vi "Program Single.vi"(8 "error in (no error)":errorcluster, 9 "Micro":string, 10 "Positions":u32, 11 "Program Driver in":refnum<class "Program Driver.lvclass">) -> (0 "error out":errorcluster, 1 "Fail Codes":string, 2 "Tests Passed":bool, 3 "Program Driver out":refnum<class "Program Driver.lvclass">)   [LabVIEW 2015, in "Program Driver.lvclass"]
uses:
  Program Driver.lvclass
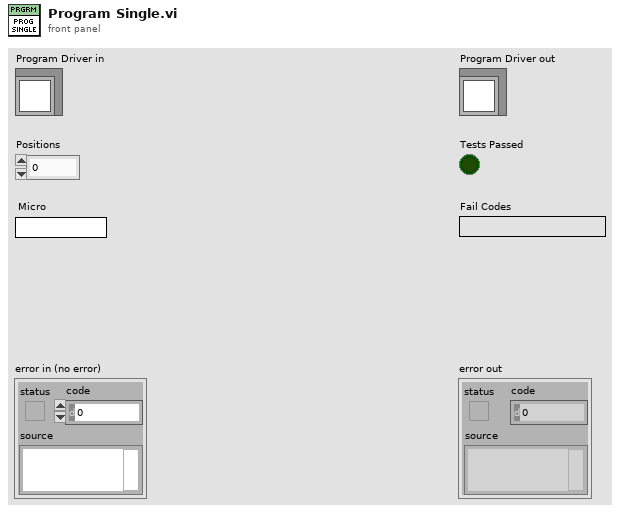
[diagram p1: front panel]
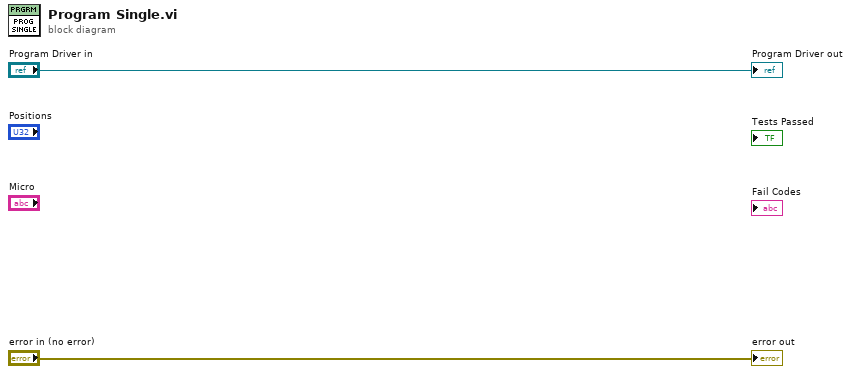
[diagram p0: block diagram]
diagram:
  "error out" <- "error in (no error)"
  "Program Driver out" <- "Program Driver in"
